vi "Get BTR wrapper.vi"(8 "error in (no error)":errorcluster caption="错误输入（无错误）", 11 "dwDevIndex":u32) -> (0 "error out":errorcluster caption="错误输出", 2 "pRtnValue out":i32, 3 "function return":u32)   [LabVIEW 2016, in "UISimCanFunc_wrapper.lvlib"]
doc: "_declspec (dllexport) DWORD GetBTR_wrapper(DWORD dwDevIndex, PINT pRtnValue);"
uses:
  <userlib>/UISimCanFunc_wrapper/UISimCanFunc_wrapper.lvlib
  <userlib>/UISimCanFunc_wrapper/UISimCanFunc_wrapper.dll
panel:
  in  "pRtnValue":i32
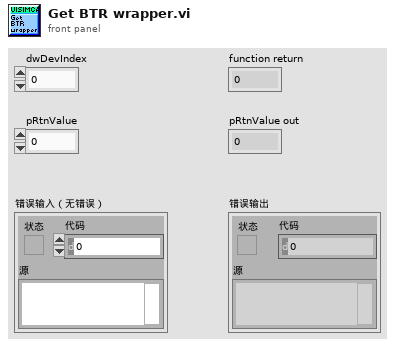
[diagram p1: front panel]
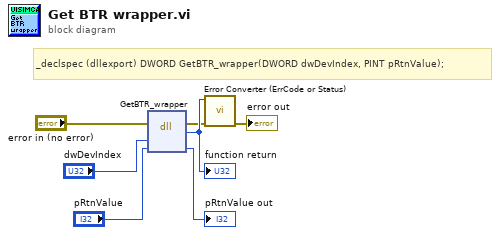
[diagram p0: block diagram]
diagram:
  # "_declspec (dllexport) DWORD GetBTR_wrapper(DWORD dwDevIndex, PINT pRtnValue);"
  n1 = dll-call lib="C:/Program Files (x86)/National Instruments/LabVIEW 2016/user.lib/UISimCanFunc_wrapper/UISimCanFunc_wrapper.*" fn="GetBTR_wrapper"(error in="error in (no error)", "dwDevIndex"="dwDevIndex", "pRtnValue"="pRtnValue") -> (error out=w2:errorcluster, w7:u32, "pRtnValue"=→"pRtnValue out":i32)  [unwired: 3 in, 1 out]
  "function return" <- w7
  n2 = call <userlib>:"Error Converter (ErrCode or Status).vi"("error in (no error)"=w2, "error code"=w7) -> ("error out"=→"error out":errorcluster)  [unwired: 9 in]
